vi "Creat Full Temperature Graph.vi"(8 "error in (no error)":errorcluster, 10 "tdms file in":refnum<k34>, 11 "NI_report in":refnum<class "NI_report.lvclass">) -> (0 "error out":errorcluster, 2 "tdms file out":refnum<k34>, 3 "NI_report out":refnum<class "NI_report.lvclass">)   [LabVIEW 2015]
uses:
  <vilib>/Utility/NIReport.llb/NI_report.lvclass
  <vilib>/Utility/NIReport.llb/Word/NI_Word.lvclass
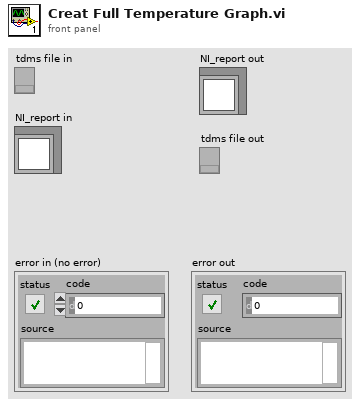
[diagram p1: front panel]
types:
  T1 = cluster{"has major gridlines?":bool, "has minor gridlines?":bool, "major gridlines color":u32, "minor gridlines color":u32}
  T2 = cluster{"font style":string, "bold":bool, "italic":bool, "underline":bool, "size":sgl, "color":u32}
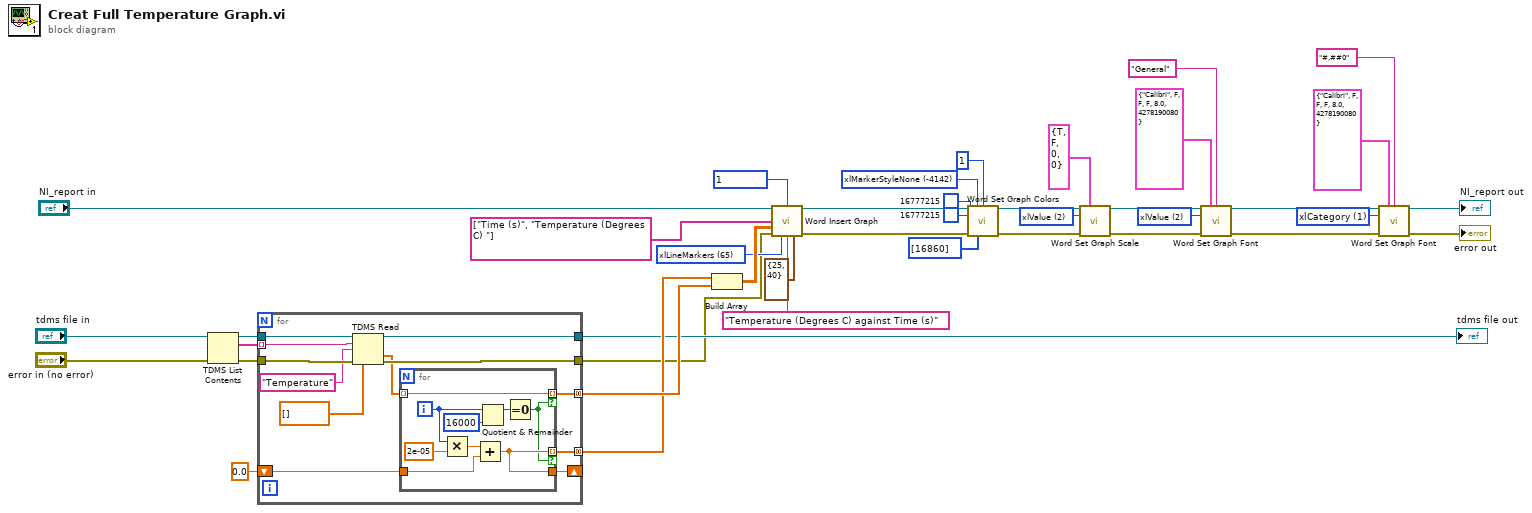
[diagram p0: block diagram]
diagram:
  w29 = 1 items=["xlCategory"=1, "xlSeriesAxis"=3, "xlValue"=2] ("axis type (category)")
  w27 = 2 items=["xlCategory"=1, "xlSeriesAxis"=3, "xlValue"=2] ("axis type (category)")
  w22 = 2 items=["xlCategory"=1, "xlSeriesAxis"=3, "xlValue"=2] ("axis type (xlCategory)")
  w17 = -4142 items=["xlMarkerStyleAutomatic"=-4105, "xlMarkerStyleCircle"=8, "xlMarkerStyleDash"=-4115, "xlMarkerStyleDiamond"=2, "xlMarkerStyleDot"=-4118, "xlMarkerStyleNone"=-4142, "xlMarkerStylePicture"=-4147, "xlMarkerStylePlus"=9, "xlMarkerStyleSquare"=1, "xlMarkerStyleStar"=5, "xlMarkerStyleTriangle"=3, "xlMarkerStyleX"=-4168] ("marker style (none)")
  w9 = 65 items=["xlColumnClustered"=51, "xlColumnStacked"=52, "xlColumnStacked100"=53, "xl3DColumnClustered"=54, "xl3DColumnStacked"=55, "xl3DColumnStacked100"=56, "xlBarClustered"=57, "xlBarStacked"=58, "xlBarStacked100"=59, "xl3DBarClustered"=60, "xl3DBarStacked"=61, "xl3DBarStacked100"=62, "xlLineStacked"=63, "xlLineStacked100"=64, "xlLineMarkers"=65, "xlLineMarkersStacked"=66, "xlLineMarkersStacked100"=67, "xlPieOfPie"=68, "xlPieExploded"=69, "xl3DPieExploded"=70, "xlBarOfPie"=71, "xlXYScatterSmooth"=72, "xlXYScatterSmoothNoMarkers"=73, "xlXYScatterLines"=74, "xlXYScatterLinesNoMarkers"=75, "xlAreaStacked"=76, "xlAreaStacked100"=77, "xl3DAreaStacked"=78, "xl3DAreaStacked100"=79, "xlDoughnutExploded"=80, "xlRadarMarkers"=81, "xlRadarFilled"=82, "xlSurface"=83, "xlSurfaceWireframe"=84, "xlSurfaceTopView"=85, "xlSurfaceTopViewWireframe"=86, "xlBubble"=15, "xlBubble3DEffect"=87, "xlStockHLC"=88, "xlStockOHLC"=89, "xlStockVHLC"=90, "xlStockVOHLC"=91, "xlCylinderColClustered"=92, "xlCylinderColStacked"=93, "xlCylinderColStacked100"=94, "xlCylinderBarClustered"=95, "xlCylinderBarStacked"=96, "xlCylinderBarStacked100"=97, "xlCylinderCol"=98, "xlConeColClustered"=99, "xlConeColStacked"=100, "xlConeColStacked100"=101, "xlConeBarClustered"=102, "xlConeBarStacked"=103, "xlConeBarStacked100"=104, "xlConeCol"=105, "xlPyramidColClustered"=106, "xlPyramidColStacked"=107, "xlPyramidColStacked100"=108, "xlPyramidBarClustered"=109, "xlPyramidBarStacked"=110, "xlPyramidBarStacked100"=111, "xlPyramidCol"=112, "xl3DColumn"=-4100, "xlLine"=4, "xl3DLine"=-4101, "xl3DPie"=-4102, "xlPie"=5, "xlXYScatter"=-4169, "xl3DArea"=-4098, "xlArea"=1, "xlDoughnut"=-4120, "xlRadar"=-4151] ("graph type (col clustered)")
  n1 = TDMS List Contents(4:"error in (no error)", 7:"tdms file in") -> (0:w4:errorcluster, 2:w1:string[], 3:w5:refnum<k34>)  [unwired: 1 in, 1 out]
  n2 = for {
    tunnel: w1 -> [w52] mode=indexing
    tunnel: w5 -> [w51]
    tunnel: w4 -> [w50]
    tunnel: [w47] -> w8
    tunnel: [w46] -> w3
    tunnel: [w44] -> w25 mode=concatenating
    tunnel: [w43] -> w24 mode=concatenating
    shift-right: [w42] -> _
    shift-left: 0.0 -> [w41]
    n3 = TDMS Read(0:w51, 5:w52, 7:"Temperature", 11:w50, 12:dbl[] []) -> (4:w47:refnum<k34>, 10:w45:dbl[], 15:w46:errorcluster)  [unwired: 3 in, 3 out]
    n4 = for {
      tunnel: w45 -> [w60] mode=indexing
      tunnel: [w60] -> w44 mode=indexing if=w53
      tunnel: [w54] -> w43 mode=indexing if=w53
      tunnel: [w54] -> w42
      tunnel: w41 -> [w55]
      i -> [w58]
      n5 = Multiply(x=w58, y=2e-05) -> (x*y=w56:dbl)
      n6 = Add(x=w56, y=w55) -> (x+y=w54:dbl)
      n7 = Quotient & Remainder(x=w58, y=16000) -> (x-y*floor(x/y)=w61:i32)  [unwired: 1 out]
      n8 = Equal To 0?(x=w61) -> (x = 0?=w53:bool)
    }
  }
  "tdms file out" <- w8
  n9 = Build Array(w24, w25) -> (w13:dbl[][])
  n10 = call <vilib>:"Word Insert Graph.vi"("report in"="NI_report in", "measurement system"=u16 1, "row headers"=string[] ["Time (s)", "Temperature (Degrees C) "] ("column headers"), "data"=w13, "error in (no error)"=w3, "graph type (col clustered)"=w9, "graph title (\"\")"="Temperature (Degrees C) against Time (s)" ("graph title (\"\")"), "graph size (5, 5)"=cluster{"height":i32, "width":i32} {"height"=25, "width"=40}) -> ("report out"=w10:refnum<class "NI_report.lvclass">, "error out"=w11:errorcluster)  [unwired: 4 in, 2 out]
  n11 = call <vilib>:"Word Set Graph Colors.vi"("report in"=w10, "marker style (none)"=w17, "weight (1)"=i16 1, "plot area color (w)"=u32 16777215, "graph area color (w)"=u32 16777215, "error in (no error)"=w11, "plot colors"=u32[] [16860]) -> ("report out"=w20:refnum<class "NI_report.lvclass">, "error out"=w21:errorcluster)  [unwired: 7 in]
  n12 = call <vilib>:"Word Set Graph Scale.vi"("report in"=w20, "gridlines"=T1 {"has major gridlines?"=TRUE, "has minor gridlines?"=FALSE, "major gridlines color"=0, "minor gridlines color"=0}, "axis type (xlCategory)"=w22, "error in (no error)"=w21) -> ("report out"=w39:refnum<class "NI_report.lvclass">, "error out"=w40:errorcluster)  [unwired: 10 in]
  n13 = call <vilib>:"Word Set Graph Font.vi"("report in"=w39, "axis font"=T2 {"font style"="Calibri", "bold"=FALSE, "italic"=FALSE, "underline"=FALSE, "size"=8.0, "color"=4278190080}, "number format (general)"="General", "axis type (category)"=w27, "error in (no error)"=w40) -> ("report out"=w32:refnum<class "NI_report.lvclass">, "error out"=w33:errorcluster)  [unwired: 9 in]
  n14 = call <vilib>:"Word Set Graph Font.vi"("report in"=w32, "axis font"=T2 {"font style"="Calibri", "bold"=FALSE, "italic"=FALSE, "underline"=FALSE, "size"=8.0, "color"=4278190080}, "number format (general)"="#,##0", "axis type (category)"=w29, "error in (no error)"=w33) -> ("report out"=→"NI_report out":refnum<class "NI_report.lvclass">, "error out"=→"error out":errorcluster)  [unwired: 9 in]
